vi "Obtain Request Events.vi"(8 "error in (no error)":errorcluster, 10 "Create New?":bool) -> (0 "error out":errorcluster, 2 "N4L_PSM3750_Interface Request Events":T1)   [LabVIEW 2025, in "N4L_PSM3750_Interface.lvlib"]
doc: "This VI Obtains/Creates the Requests events that will be used for other modules to communicate with the module that owns this VI. These Requests events will be accessed only via Public API methods for this module.\n\n<b>NOTE</b>: The contents of this VI are automatically generated and modified by the <b>Tools > Delacor > DQMH</b> utilities. Consider using those utilities instead of making your own modifications to this VI.\n_____\nBased on Delacor QMH Project Template 3.1.0.34."
uses:
  N4L_PSM3750_Interface.lvlib
  Request Events--cluster.ctl
  Stop Argument--cluster.ctl
  Show Panel Argument--cluster.ctl
  Hide Panel Argument--cluster.ctl
  Get Module Execution Status Argument--cluster.ctl
  Show Diagram Argument--cluster.ctl
  Change Panel Argument--cluster.ctl
  <vilib>/MGI/Panel Manager/Panel/Panel/Panel.lvclass
  Initialise N4L Connection Argument--cluster.ctl
  Initialise--cluster.ctl
  Close N4L Connection Argument--cluster.ctl
  Reset N4L Instrument Argument--cluster.ctl
  Set Generator Configuration Argument--cluster.ctl
  Generator Config--cluster.ctl
  Set Generator Output Argument--cluster.ctl
  Set Range Argument--cluster.ctl
  Range Config--cluster.ctl
  Set Trim Configuration Argument--cluster.ctl
panel:
  # "NOTE: The contents of this VI are automatically generated and modified by the Tools > Delacor > DQMH utilities. Consider using those utilities instead of making your own modifications to this VI."
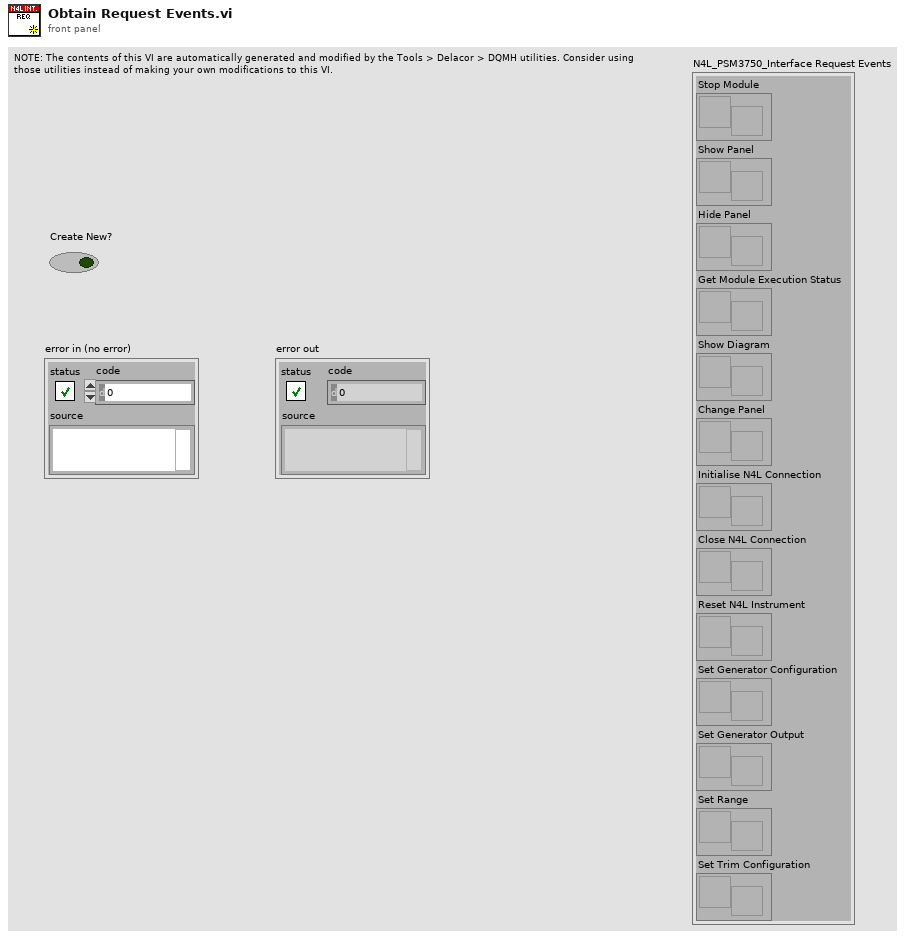
[diagram p1: front panel]
types:
  T1 = typedef "N4L_PSM3750_Interface.lvlib/Request Events--cluster.ctl" = cluster{"Stop Module":refnum<user-event>, "Show Panel":refnum<user-event>, "Hide Panel":refnum<user-event>, "Get Module Execution Status":refnum<user-event>, "Show Diagram":refnum<user-event>, "Change Panel":refnum<user-event>, "Initialise N4L Connection":refnum<user-event>, "Close N4L Connection":refnum<user-event>, "Reset N4L Instrument":refnum<user-event>, "Set Generator Configuration":refnum<user-event>, "Set Generator Output":refnum<user-event>, "Set Range":refnum<user-event>, "Set Trim Configuration":refnum<user-event>}
  T2 = typedef "N4L_PSM3750_Interface.lvlib/Set Trim Configuration Argument--cluster.ctl" = cluster{"Set Trim Config":cluster{"AC Trim Data (Disabled)":u16, "AC Level (1)":dbl, "Tolerance (10)":dbl}}
  T3 = typedef "N4L_PSM3750_Interface.lvlib/Set Range Argument--cluster.ctl" = cluster{"Range":T4}
  T4 = typedef "N4L_PSM3750_Interface.lvlib/Range Config--cluster.ctl" = cluster{"Input Ranging Mode (Auto)":enum16{"AUTO", "UPAUTO", "1mV", "3mV", "10mV", "30mV", "100mV", "300mV", "1V", "3V", "10V"}, "Input Input Type (Internal)":u16, "Input Selection (CH1)":enum16{"CH1", "CH2"}, "Input Connection (Main) ":u16, "Input Coupling (Internal)":enum16{"AC+DC", "AC"}, "Input Shunt Value (0,02)":dbl, "Input Voltage Scale factor (1)":dbl}
  T5 = typedef "N4L_PSM3750_Interface.lvlib/Set Generator Output Argument--cluster.ctl" = cluster{"Generator Output":enum16{"OFF", "ON"}}
  T6 = typedef "N4L_PSM3750_Interface.lvlib/Set Generator Configuration Argument--cluster.ctl" = cluster{"Generator Configuration":T7}
  T7 = typedef "N4L_PSM3750_Interface.lvlib/Generator Config--cluster.ctl" = cluster{"Waveform":enum16{"Sinewave", "Square"}, "Frequency (1000)":dbl, "Amplitude (2)":dbl, "Offset (0)":dbl}
  T8 = typedef "N4L_PSM3750_Interface.lvlib/Reset N4L Instrument Argument--cluster.ctl" = cluster{"Boolean":bool}
  T9 = typedef "N4L_PSM3750_Interface.lvlib/Close N4L Connection Argument--cluster.ctl" = cluster{"Boolean":bool}
  T10 = typedef "N4L_PSM3750_Interface.lvlib/Initialise N4L Connection Argument--cluster.ctl" = cluster{"N4L Initialise":T11}
  T11 = typedef "N4L_PSM3750_Interface.lvlib/Initialise--cluster.ctl" = cluster{"VISA resource name":refnum<visa-resource-name>, "Baud Rate":u32, "ID Query":bool, "Reset":bool}
  T12 = typedef "N4L_PSM3750_Interface.lvlib/Change Panel Argument--cluster.ctl" = cluster{"New Panel":refnum<class "Panel.lvclass">}
  T13 = typedef "N4L_PSM3750_Interface.lvlib/Hide Panel Argument--cluster.ctl" = cluster{"Hide Panel?":bool}
  T14 = typedef "N4L_PSM3750_Interface.lvlib/Show Panel Argument--cluster.ctl" = cluster{"Show Panel?":bool}
  T15 = typedef "N4L_PSM3750_Interface.lvlib/Show Diagram Argument--cluster.ctl" = cluster{"Debug?":bool}
  T16 = typedef "N4L_PSM3750_Interface.lvlib/Get Module Execution Status Argument--cluster.ctl" = cluster{"Running?":bool}
  T17 = typedef "N4L_PSM3750_Interface.lvlib/Stop Argument--cluster.ctl" = cluster{"Origin":string, "Exit via Stop Module Req?":bool, "Wait for Module to stop?":bool}
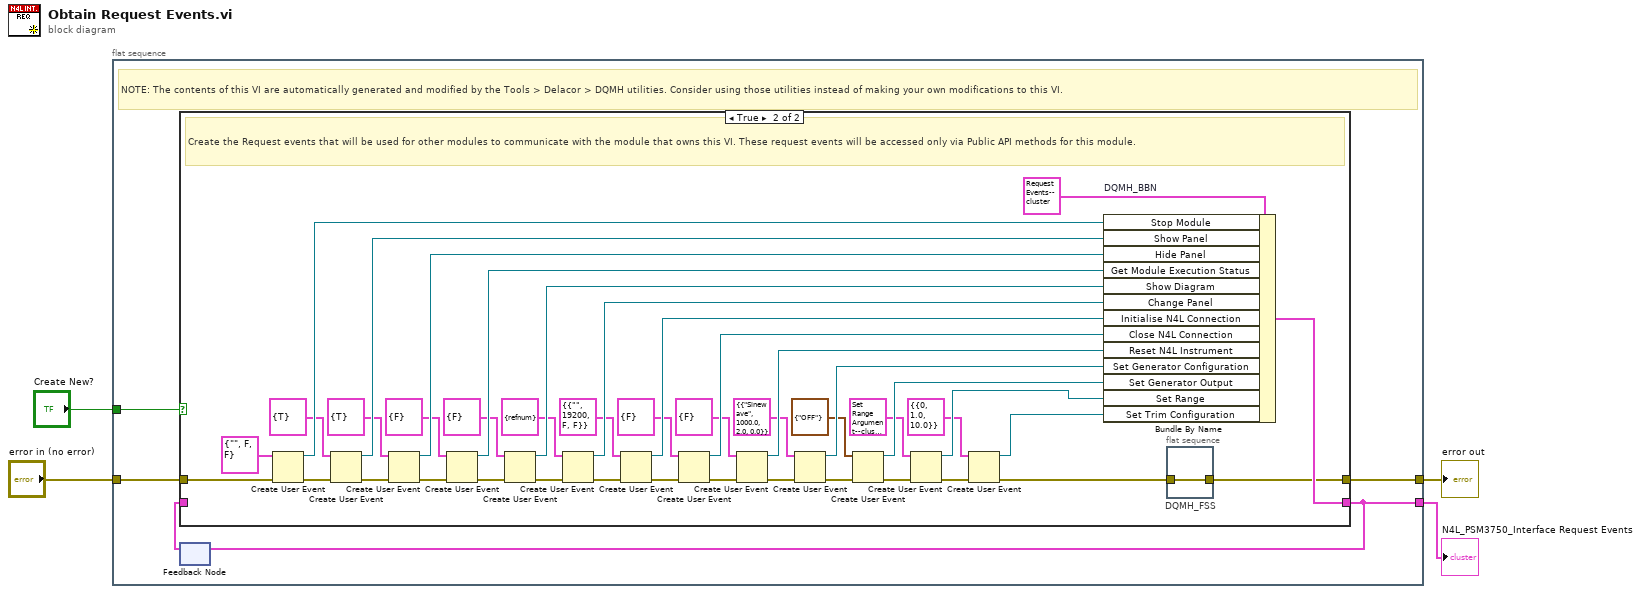
[diagram p0: block diagram]
diagram:
  n1 = flat-sequence {
    tunnel: [w9] -> w4
    tunnel: "error in (no error)" -> [w8]
    tunnel: [w6] -> w2
    tunnel: "Create New?" -> [w5]
    frame #0 {
      # "NOTE: The contents of this VI are automatically generated and modified by the Tools > Delacor > DQMH utilities. Consider using those utilities instead of making your own modifications to this VI."
      n2 = feedback #1() -> (w7:T1)  [unwired: 1 in]
      n3 = case shown="True" w5 {
        tunnel: [w10 w44] -> w9
        tunnel: w8 -> [w10 w54]
        tunnel: [w11 w51] -> w6
        tunnel: w7 -> [w11 _]
        frame False {
          # "Obtain the Request events that were created in a previous call to this VI."
        }
        frame True {
          # "Create the Request events that will be used for other modules to communicate with the module that owns this VI. These request events will be accessed only via Public API methods for this module."
          n4 = Create User Event(user event datatype=T17 {"Origin"="", "Exit via Stop Module Req?"=FALSE, "Wait for Module to stop?"=FALSE} ("Stop Argument"), error in=w54) -> (user event=w52:refnum<user-event>, error out=w49:errorcluster)
          n5 = Create User Event(user event datatype=T14 {"Show Panel?"=TRUE} ("Show Panel Argument"), error in=w49) -> (user event=w48:refnum<user-event>, error out=w47:errorcluster)
          n6 = Create User Event(user event datatype=T13 {"Hide Panel?"=TRUE} ("Hide Panel Argument"), error in=w47) -> (user event=w46:refnum<user-event>, error out=w45:errorcluster)
          n7 = Create User Event(user event datatype=T16 {"Running?"=FALSE} ("Get Module Execution Status Argument"), error in=w45) -> (user event=w42:refnum<user-event>, error out=w43:errorcluster)
          n8 = Create User Event(user event datatype=T15 {"Debug?"=FALSE} ("Show Diagram Argument"), error in=w43) -> (user event=w39:refnum<user-event>, error out=w40:errorcluster)
          n9 = Create User Event(user event datatype=T12 {"New Panel"=refnum} ("Change Panel Argument"), error in=w40) -> (user event=w34:refnum<user-event>, error out=w35:errorcluster)
          n10 = Create User Event(user event datatype=T10 {"N4L Initialise"={"VISA resource name"="", "Baud Rate"=19200, "ID Query"=FALSE, "Reset"=FALSE}} ("Initialise N4L Connection Argument"), error in=w35) -> (user event=w31:refnum<user-event>, error out=w32:errorcluster)
          n11 = Create User Event(user event datatype=T9 {"Boolean"=FALSE} ("Close N4L Connection Argument"), error in=w32) -> (user event=w28:refnum<user-event>, error out=w29:errorcluster)
          n12 = Create User Event(user event datatype=T8 {"Boolean"=FALSE} ("Reset N4L Instrument Argument"), error in=w29) -> (user event=w25:refnum<user-event>, error out=w26:errorcluster)
          n13 = Create User Event(user event datatype=T6 {"Generator Configuration"={"Waveform"=enum."Sinewave", "Frequency (1000)"=1000.0, "Amplitude (2)"=2.0, "Offset (0)"=0.0}} ("Set Generator Configuration Argument"), error in=w26) -> (user event=w22:refnum<user-event>, error out=w23:errorcluster)
          n14 = Create User Event(user event datatype=T5 {"Generator Output"=enum."OFF"} ("Set Generator Output Argument"), error in=w23) -> (user event=w19:refnum<user-event>, error out=w20:errorcluster)
          n15 = Create User Event(user event datatype=T3 {"Range"={"Input Ranging Mode (Auto)"=enum."AUTO", "Input Input Type (Internal)"=1, "Input Selection (CH1)"=enum."CH1", "Input Connection (Main) "=0, "Input Coupling (Internal)"=enum."AC+DC", "Input Shunt Value (0,02)"=0.02, "Input Voltage Scale factor (1)"=1.0}} ("Set Range Argument"), error in=w20) -> (user event=w16:refnum<user-event>, error out=w17:errorcluster)
          n16 = Create User Event(user event datatype=T2 {"Set Trim Config"={"AC Trim Data (Disabled)"=0, "AC Level (1)"=1.0, "Tolerance (10)"=10.0}} ("Set Trim Configuration Argument"), error in=w17) -> (user event=w13:refnum<user-event>, error out=w14:errorcluster)
          n17 = Bundle By Name "DQMH_BBN"(cluster=T1 {"Stop Module"=refnum, "Show Panel"=refnum, "Hide Panel"=refnum, "Get Module Execution Status"=refnum, "Show Diagram"=refnum, "Change Panel"=refnum, "Initialise N4L Connection"=refnum, "Close N4L Connection"=refnum, "Reset N4L Instrument"=refnum, "Set Generator Configuration"=refnum, "Set Generator Output"=refnum, "Set Range"=refnum, "Set Trim Configuration"=refnum} ("output cluster"), "Stop Module"=w52, "Show Panel"=w48, "Hide Panel"=w46, "Get Module Execution Status"=w42, "Show Diagram"=w39, "Change Panel"=w34, "Initialise N4L Connection"=w31, "Close N4L Connection"=w28, "Reset N4L Instrument"=w25, "Set Generator Configuration"=w22, "Set Generator Output"=w19, "Set Range"=w16, "Set Trim Configuration"=w13) -> (w51:T1)
          n18 = flat-sequence "DQMH_FSS" {
            tunnel: w14 -> [w55]
            tunnel: [w55] -> w44
            frame #0 {
            }
          }
        }
      }
      n19 = feedback-in #1(w6) -> ()
    }
  }
  "N4L_PSM3750_Interface Request Events" <- w2
  "error out" <- w4
